vi "eventHandler.vi"(0 "Boolean in":refnum<vi>, 1 "label":string, 5 "Sub Panel 2":refnum<vi>, 9 "Sub Panel":refnum<vi>, 11 "event data in":T1) -> (15 "event data out":T1)   [LabVIEW 2020]
uses:
  Controls/eventtypdef1.ctl
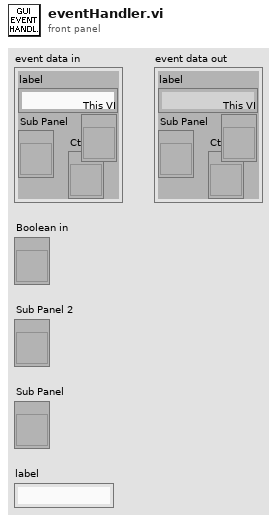
[diagram p1: front panel]
types:
  T1 = typedef "eventtypdef1.ctl" = cluster{"label":string, "Sub Panel":refnum<vi>, "CtlRef":refnum<vi>, "This VI":refnum<vi>}
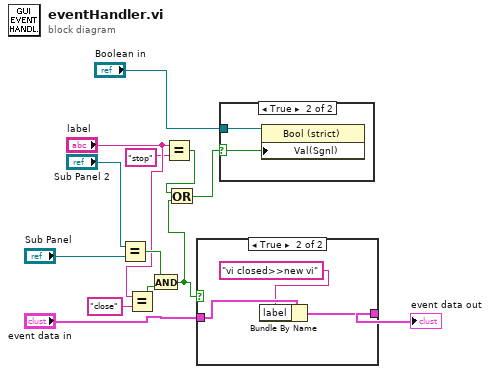
[diagram p0: block diagram]
diagram:
  n1 = Equal?(x="Sub Panel 2", y="Sub Panel") -> (x = y?=w11:bool)
  n2 = Equal?(x="label", y="close") -> (x = y?=w12:bool)
  n3 = And(x=w11, y=w12) -> (x .and. y?=w13:bool)
  n4 = Equal?(x="label", y="stop") -> (x = y?=w7:bool)
  n5 = Or(x=w7, y=w13) -> (x .or. y?=w8:bool)
  n6 = case shown="True" w13 {
    tunnel: "event data in" -> [w14 w17]
    tunnel: [w14 w16] -> w6
    frame False {
    }
    frame True {
      n7 = Bundle By Name(cluster=w17, "label"="vi closed>>new vi") -> (w16:T1)
    }
  }
  "event data out" <- w6
  n8 = case shown="True" w8 {
    selector: w8 -> [_ w18]
    tunnel: "Boolean in" -> [_ w19]
    frame False {
    }
    frame True {
      n9 = property class="Bool (strict)"(reference=w19, "Val(Sgnl)"=w18) -> ()  [unwired: 1 in, 2 out]
    }
  }
